vi "Smart IO Set Digital Output.vi"(8 "error in (no error)":errorcluster, 10 "value":bool, 11 "deviceIndex":i32) -> (0 "error out":errorcluster)   [LabVIEW 2026, in "MrcLib.lvlib"]
doc: "Update the output pin of the selected device channel to low or high digital voltage value."
uses:
  MrcLib.lvlib
  Types/MRC Smart IO Mode.ctl
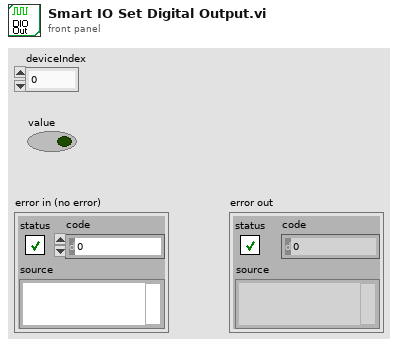
[diagram p1: front panel]
types:
  T1 = typedef "MRC Smart IO Mode.ctl" = i32
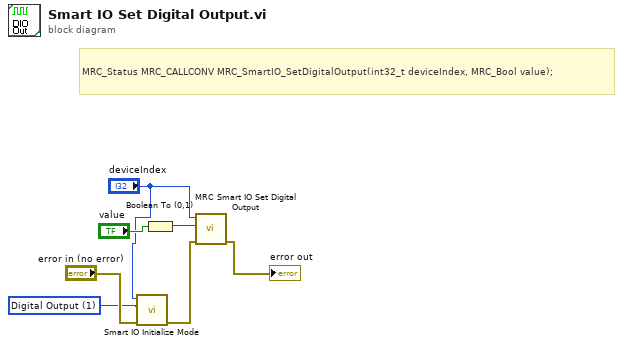
[diagram p0: block diagram]
diagram:
  w1 = T1 1 items=["Digital Input"=0, "Digital Output"=1, "Analog Input"=2, "PWM Input"=3, "PWM Output"=4, "Counter Rising"=5, "Counter Falling"=6, "Addressable LEDs"=13] ("mode")
  # "MRC_Status MRC_CALLCONV MRC_SmartIO_SetDigitalOutput(int32_t deviceIndex, MRC_Bool value);"
  n1 = call "Smart IO Initialize Mode.vi"("error in (no error)"="error in (no error)", "mode"=w1, "deviceIndex"="deviceIndex") -> ("error out"=w4:errorcluster)  [unwired: 8 in]
  n2 = Boolean To (0,1)(Boolean="value") -> (0, 1=w6:i16)
  n3 = call "MRC Smart IO Set Digital Output.vi"("error in (no error)"=w4, "value"=w6, "deviceIndex"="deviceIndex") -> ("error out"=→"error out":errorcluster)  [unwired: 8 in]
